vi "GetWindowMouseRect.vi"(8 "No Error":errorcluster, 11 "Window [SDL_Window *]":T2 format="%.0x") -> (0 "Error Out":errorcluster, 2 "Has Confinement Rectangle?":bool, 3 "Rect":T1)   [LabVIEW 2026, in "SDL3.lvlib" / "Video.lvlib"]
doc: "<B>Summary</B>\nGet the mouse confinement rectangle of a window."
uses:
  Video.lvlib
  Rect/Rect--cluster.ctl
  Rect/Rect.lvlib
  Lib/SDL3.dll
  SDL_Window--pointer.ctl
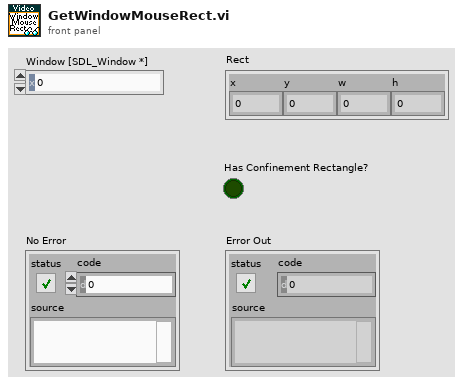
[diagram p1: front panel]
types:
  T1 = typedef "SDL3.lvlib/Rect.lvlib/Rect--cluster.ctl" = cluster{"x":i32, "y":i32, "w":i32, "h":i32}
  T2 = typedef "SDL3.lvlib/Video.lvlib/SDL_Window--pointer.ctl" = i64
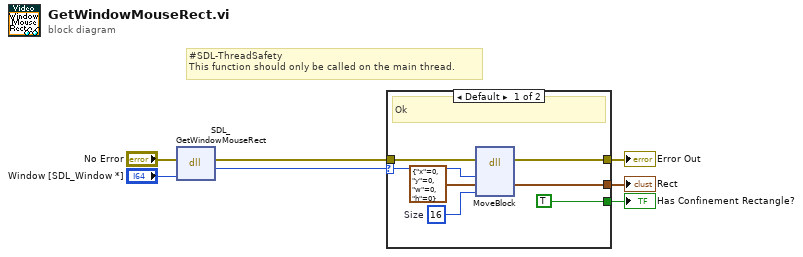
[diagram p0: block diagram]
diagram:
  # "#SDL-ThreadSafety\nThis function should only be called on the main thread."
  n1 = dll-call lib="C:/Users/saukko/Dev/LV-SDL3/Sources/SDL3/Lib/SDL3.*" fn="SDL_GetWindowMouseRect"(error in="No Error", "window"="Window [SDL_Window *]") -> (error out=w5:errorcluster, "return type"=w4:i64)  [unwired: 3 in, 1 out]
  n2 = case shown="Default" w4 {
    selector: w4 -> [w13 _]
    tunnel: w5 -> [w14 w15]
    tunnel: [w8 w15] -> w3
    tunnel: [w10 _] -> w2
    tunnel: [TRUE ("Has Confinement Rectangle?") _] -> w1
    frame Default {
      w11 = 16  # Size
      # "Ok"
      n3 = dll-call lib="LabVIEW" fn="MoveBlock"(error in=w14, "Address"=w13, "Destination"=T1 {"x"=0, "y"=0, "w"=0, "h"=0} ("Rect"), "Size"=w11) -> (error out=w8:errorcluster, "Destination"=w10:T1)  [unwired: 5 in, 1 out]
    }
    frame 0 {
      # "No confinement rectangle"
    }
  }
  "Error Out" <- w3
  "Rect" <- w2
  "Has Confinement Rectangle?" <- w1
